vi "LVClasse_SurfaceFloatWithPupil dtor.vi"(0 "SurfaceFloatWithPupil in":refnum<class "SurfaceFloatWithPupil.lvclass">, 11 "error in (no error)":errorcluster) -> (4 "SurfaceFloatWithPupil out":refnum<class "SurfaceFloatWithPupil.lvclass">, 15 "error out":errorcluster)   [LabVIEW 2020, in "SurfaceFloatWithPupil.lvclass"]
doc: "Phase destructor.\n\n--------------------------------------------------------------------------------\n\n<B>PhaseIn</B> : Phase object.\n<B>PhaseOut</B> : Phase object.\n<B>ErrorIn</B> : Error\n<B>ErrorOut</B> : Error\n\n--------------------------------------------------------------------------------"
uses:
  SurfaceFloatWithPupil.lvclass
  SurfaceFloatWithPupil.lvclass/SurfaceFloatWithPupil.ctl
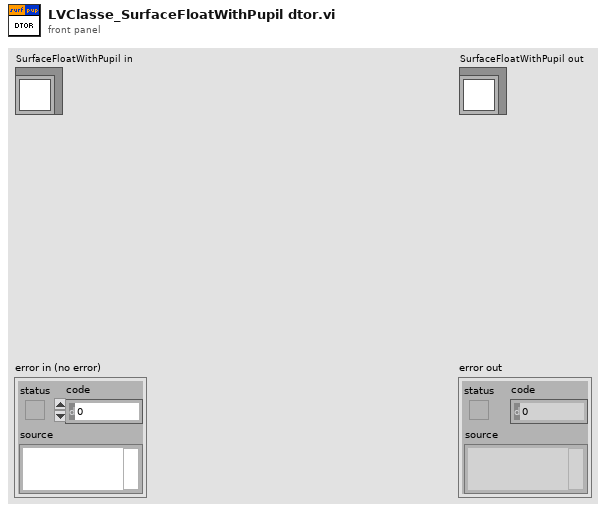
[diagram p1: front panel]
types:
  T1 = typedef "Handle creation.ctl" = enum16{"By ctor", "By write function"}
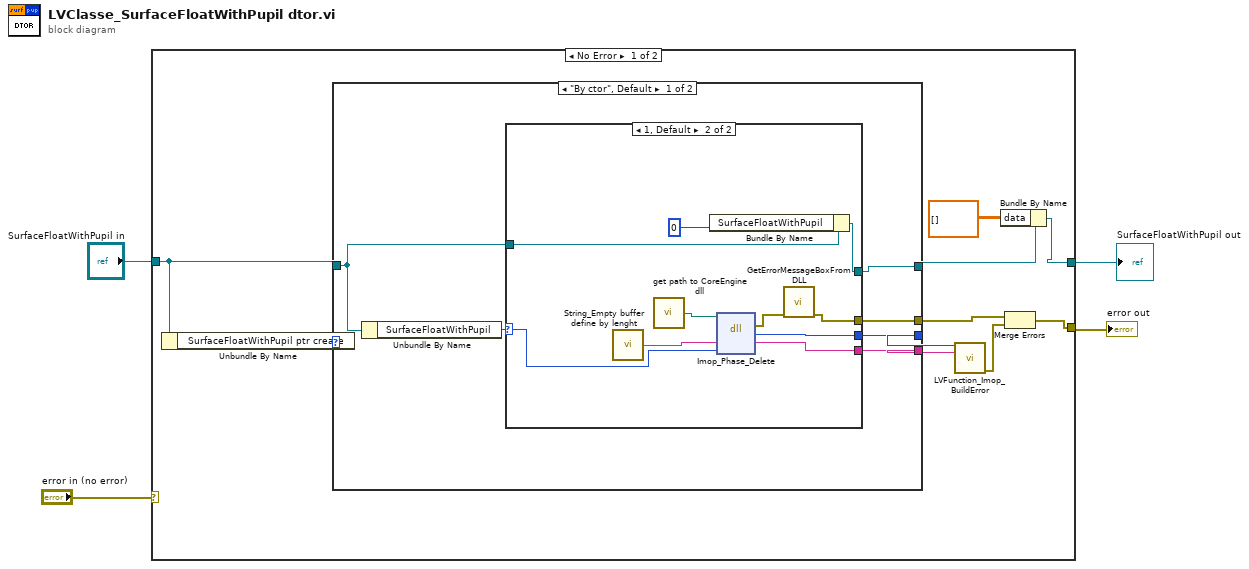
[diagram p0: block diagram]
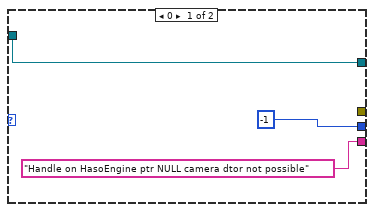
[diagram p2: hidden frame]
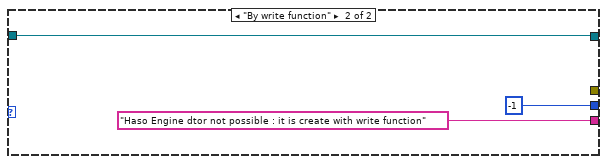
[diagram p3: hidden frame]
diagram:
  n1 = case shown="No Error" "error in (no error)" {
    selector: "error in (no error)" -> [_ w37]
    tunnel: "SurfaceFloatWithPupil in" -> [w12 w38]
    tunnel: [w6 w38] -> w2
    tunnel: [w8 w37] -> w1
    frame No Error {
      n2 = Unbundle By Name(w12) -> ("SurfaceFloatWithPupil ptr create"=w11:T1)
      n3 = case shown="\"By ctor\", Default" w11 {
        tunnel: [w20 "Haso Engine dtor not possible : it is create with write function" ("message")] -> w14
        tunnel: [w19 -1] -> w13
        tunnel: w12 -> [w17 w34]
        tunnel: [w18 w34] -> w7
        tunnel: [w15 _] -> w10
        frame "By ctor", Default {
          n4 = Unbundle By Name(w17) -> ("SurfaceFloatWithPupil"=w16:i32)
          n5 = case shown="1, Default" w16 {
            selector: w16 -> [_ w30]
            tunnel: ["Handle on HasoEngine ptr NULL camera dtor not possible" ("message") w32] -> w20
            tunnel: [-1 w31] -> w19
            tunnel: w17 -> [w21 w26]
            tunnel: [w21 w25] -> w18
            tunnel: [_ w24] -> w15
            frame 0 {
            }
            frame 1, Default {
              n6 = call "String_Empty buffer define by lenght.vi"() -> ("Empty buffer"=w33:string)  [unwired: 1 in]
              n7 = call "get path to CoreEngine dll.vi"() -> ("path to c_interface_vc100.dll"=w29:path)  [unwired: 12 in, 3 out]
              n8 = Bundle By Name(cluster=w26, "SurfaceFloatWithPupil"=u32 0 ("HasoEgine")) -> (w25:refnum<class "SurfaceFloatWithPupil.lvclass">)
              n9 = dll-call lib="D:/soft/HASO_v3/SVN_trunk/ImOpCoreEngine4_LV2011/DLLs/c_interface_vc100.dll" fn="Imop_Phase_Delete"(path in=w29, "message"=w33, "objet"=w30) -> (error out=w28:errorcluster, "return type"=w31:i32, "message"=w32:string)  [unwired: 3 in, 1 out]
              n10 = call "GetErrorMessageBoxFromDLL.vi"("error IN"=w28) -> ("error OUT"=w24:errorcluster)  [unwired: 10 in]
            }
          }
        }
        frame "By write function" {
        }
      }
      n11 = call "LVFunction_Imop_BuildError.vi"("code"=w13, "String to Prepend to source (\"\")"=w14) -> ("error out"=w9:errorcluster)  [unwired: 13 in]
      n12 = Bundle By Name(cluster=w7, "data"=sgl[][] []) -> (w6:refnum<class "SurfaceFloatWithPupil.lvclass">)
      n13 = Merge Errors(w10, w9) -> (w8:errorcluster)
    }
    frame Error {
    }
  }
  "error out" <- w1
  "SurfaceFloatWithPupil out" <- w2
